vi "Delete COMPOSER Gas Mix.vi"(7 "Unit ID (A)":string="A", 8 "error in":errorcluster, 9 "Gas Number":u16=236 min=236 max=255, 11 "VISA Session In":refnum<visa-resource-name>="Alicat") -> (0 "error out":errorcluster, 3 "VISA Session Out":refnum<visa-resource-name>)   [LabVIEW 2015]
doc: "Deletes a custom COMPOSER gas mix based on the specified gas number. Valid gas numbers for COMPOSER gases are 236-255."
uses:
  <vilib>/Instr/_visa.llb/VISA Flush IO Buffer Mask.ctl
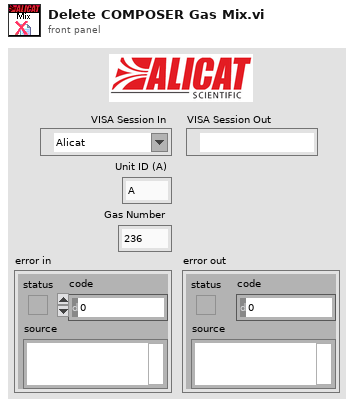
[diagram p1: front panel]
types:
  T1 = typedef "VISA Flush IO Buffer Mask.ctl" = u16
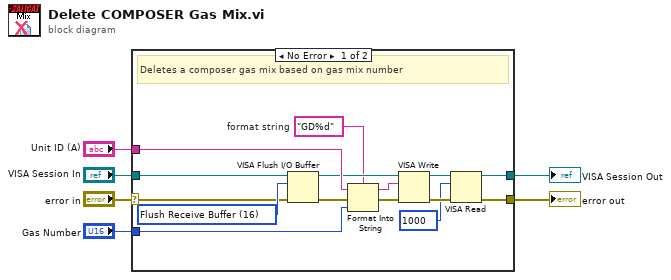
[diagram p0: block diagram]
diagram:
  n1 = case shown="No Error" "error in" {
    selector: "error in" -> [w7 w23]
    tunnel: "VISA Session In" -> [w21 w22]
    tunnel: [w20 w22] -> w5
    tunnel: [w19 w23] -> w4
    tunnel: "Unit ID (A)" -> [w18 _]
    tunnel: "Gas Number" -> [w8 _]
    frame No Error {
      w9 = T1 16 items=["Flush Receive Buffer"=16, "Write Transmit Buffer to Device"=32, "Flush Receive Buffer (No I/O)"=64, "Flush Transmit Buffer"=128] ("Mask")
      w14 = "GD%d"  # format string
      # "Deletes a composer gas mix based on gas mix number"
      n2 = VISA Flush I/O Buffer(VISA resource name=w21, mask (16)=w9, error in (no error)=w7) -> (VISA resource name out=w16:refnum<visa-resource-name>, error out=w12:errorcluster)
      n3 = Format Into String(format string=w14, initial string=w18, error in=w12, w8) -> (resulting string=w13:string, error out=w11:errorcluster)
      n4 = VISA Write(VISA resource name=w16, write buffer=w13, error in (no error)=w11) -> (VISA resource name out=w15:refnum<visa-resource-name>, error out=w17:errorcluster)  [unwired: 1 out]
      n5 = VISA Read(VISA resource name=w15, byte count=u32 1000, error in (no error)=w17) -> (VISA resource name out=w20:refnum<visa-resource-name>, error out=w19:errorcluster)  [unwired: 2 out]
    }
    frame Error {
    }
  }
  "error out" <- w4
  "VISA Session Out" <- w5
